vi "CTRE_Phoenix_Pigeon2_GetGravityVector.vi"(8 "error in (no error)":errorcluster, 11 "PigeonIMUDevRef 2":T1={"DeviceStatus"={"status"=FALSE, "code"=0, "source"=""}, "Device Number"=0, "Type"=352321536, "Device ID"=0, "Handle"=0, "UsageFrame"=0, "Library Path"=path ""} {"Type" items=["CAN"=352321536, "TalonSRX"=33554432]}) -> (0 "error out":errorcluster, 2 "Gravity Vector":cluster{"X":dbl, "Y":dbl, "Z":dbl}, 3 "PigeonIMUDevRef":T1={"DeviceStatus"={"status"=FALSE, "code"=0, "source"=""}, "Device Number"=0, "Type"=352321536, "Device ID"=0, "Handle"=0, "UsageFrame"=0, "Library Path"=path ""} {"Type" items=["CAN"=352321536, "TalonSRX"=33554432]})   [LabVIEW 2020]
doc: "Gets the Gravity Vector from a Pigeon2."
uses:
  <vilib>/Rock Robotics/WPI/ThirdParty/Phoenix-LabVIEW/Pigeon IMU/CTRE_PigeonIMU_DeviceRef.ctl
  <vilib>/Rock Robotics/WPI/ThirdParty/Phoenix-LabVIEW/Pigeon IMU/CTRE_PigeonIMU_ConnectionType.ctl
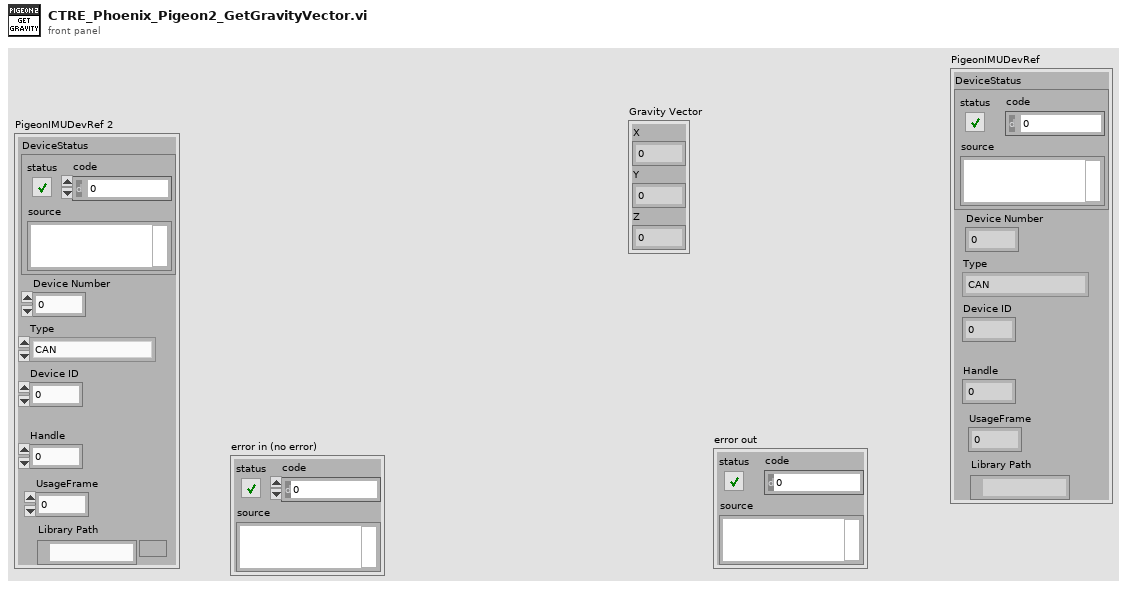
[diagram p1: front panel]
types:
  T1 = typedef "CTRE_PigeonIMU_DeviceRef.ctl" = cluster{"DeviceStatus":errorcluster, "Device Number":u8, "Type":T2, "Device ID":u32, "Handle":u64, "UsageFrame":u32, "Library Path":path}
  T2 = typedef "CTRE_PigeonIMU_ConnectionType.ctl" = u32
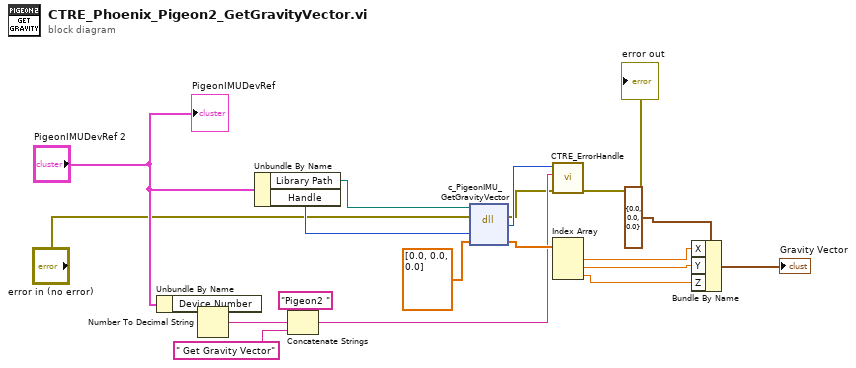
[diagram p0: block diagram]
diagram:
  n1 = Unbundle By Name("PigeonIMUDevRef 2") -> ("Device Number"=w11:u8)
  n2 = Number To Decimal String(number=w11) -> (decimal integer string=w10:string)  [unwired: 1 in]
  n3 = Unbundle By Name("PigeonIMUDevRef 2") -> ("Library Path"=w19:path, "Handle"=w18:u64)
  n4 = Concatenate Strings("Pigeon2 " ("string"), w10, " Get Gravity Vector" ("string")) -> (w6:string)
  n5 = dll-call lib="?" fn="c_PigeonIMU_GetGravityVector"(path in=w19, error in="error in (no error)", "handle"=w18, "xyz"=dbl[] [0.0, 0.0, 0.0] ("ypr")) -> (error out=w1:errorcluster, "return type"=w5:i32, "xyz"=w17:dbl[])  [unwired: 2 in, 1 out]
  n6 = call <vilib>:"CTRE_ErrorHandle.vi"("error in"=w1, "origin"=w6, "code"=w5) -> ("error out"=→"error out":errorcluster)  [unwired: 8 in]
  n7 = Index Array(array=w17) -> (element #1=w16:dbl, element #2=w15:dbl, element #3=w14:dbl)  [unwired: 3 in]
  n8 = Bundle By Name(cluster=cluster{"X":dbl, "Y":dbl, "Z":dbl} {"X"=0.0, "Y"=0.0, "Z"=0.0} ("Gravity"), "X"=w16, "Y"=w15, "Z"=w14) -> (→"Gravity Vector":cluster{"X":dbl, "Y":dbl, "Z":dbl})
  "PigeonIMUDevRef" <- "PigeonIMUDevRef 2"
